vi "Initialise.vi"(8 "error in (no error)":errorcluster, 10 "Message in":refnum<class "InitialiseMessage.lvclass">, 11 "DAQCascade512 in":refnum<class "DAQCascade512.lvclass">) -> (0 "error out":errorcluster, 3 "DAQCascade512 out":refnum<class "DAQCascade512.lvclass">)   [LabVIEW 2012, in "DAQCascade512.lvclass"]
doc: "This method is called when an initialise message is received. It mainly initialises the RabbitMQ connectivity. \n\nOverride this method when your component needs special initialisation (e.g. of software or hardware resources). In that case, don't forget to call the parent for proper implementation. If your component owns subcomponents, they count as resources, so you have to initialise them by calling their own initialise functions"
uses:
  DAQCascade512.lvclass
  <vilib>/Distrio/Murmex/InitialiseMessage/InitialiseMessage.lvclass
  <vilib>/Distrio/Murmex/Murmex/Murmex.lvclass
  DAQCascade512.lvclass/DAQCascade512.ctl
panel:
  # "This method is called when the INTIALISE\ntrigger is sent. \n\nOverride this method when your component needs to\nrespond to this trigger. \n\nCall parent for proper implementation"
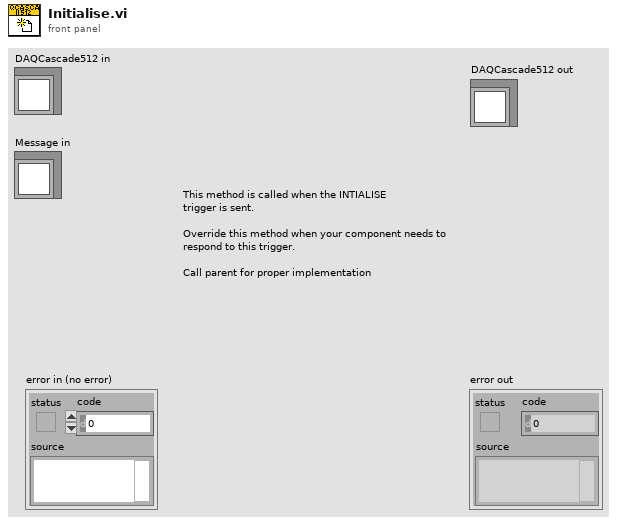
[diagram p1: front panel]
types:
  T1 = typedef "Image_type.ctl" = u32
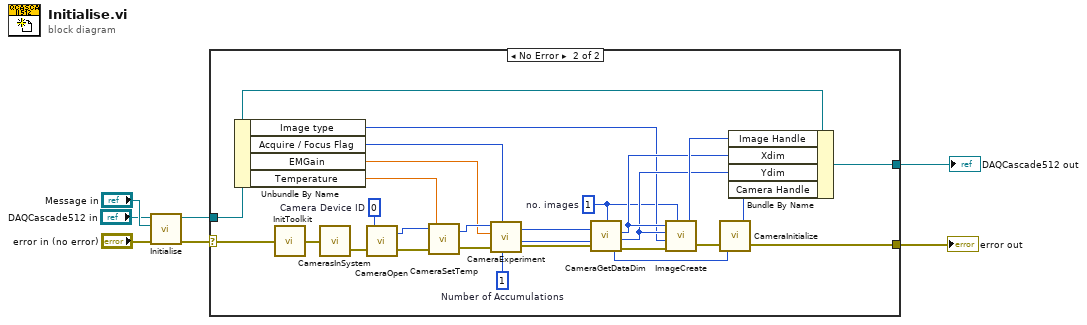
[diagram p0: block diagram]
diagram:
  n1 = call-parent "Initialise.vi"("error in (no error)"="error in (no error)", "Message in"="Message in", "Murmex in"="DAQCascade512 in") -> ("error out"=w4:errorcluster, "Murmex out"=w2:refnum<class "DAQCascade512.lvclass">)  [unwired: 7 in]
  n2 = case shown="No Error" w4 {
    selector: w4 -> [w9 w15]
    tunnel: [w9 w14] -> w3
    tunnel: w2 -> [w8 w13]
    tunnel: [w8 w11] -> w1
    frame Error {
    }
    frame No Error {
      w10 = 1  # no. images
      w29 = u32 1  # Number of Accumulations
      w35 = u32 0  # Camera Device ID
      n3 = Unbundle By Name(w13) -> ("Image type"=w16:T1, "Acquire / Focus Flag"=w17:u32, "EMGain"=w18:dbl, "Temperature"=w19:dbl)
      n4 = call <userlib>:"InitToolkit.vi"("error in"=w15) -> ("error out"=w25:errorcluster)
      n5 = call <userlib>:"CamerasInSystem.vi"("error in"=w25) -> ("error out"=w30:errorcluster)  [unwired: 1 out]
      n6 = call <userlib>:"CameraOpen.vi"("error in"=w30, "Camera Device ID"=w35) -> ("error out"=w33:errorcluster, "Camera Handle"=w34:u32)
      n7 = call <userlib>:"CameraSetTemp.vi"("error in (no error)"=w33, "Temperature"=w19, "Camera Handle"=w34) -> ("error out"=w24:errorcluster, "Camera Handle"=w23:u32)
      n8 = call <userlib>:"CameraExperiment.vi"("Number of Accumulations"=w29, "Acquire / Focus Flag"=w17, "error in"=w24, "Number of Images"=w10, "Exposure (sec)"=w18, "Camera Handle"=w23) -> ("error out"=w32:errorcluster, "Camera Handle"=w27:u32)
      n9 = call <userlib>:"CameraGetDataDim.vi"("Camera Handle"=w27, "error in"=w32) -> ("Camera Handle"=w26:u32, "Xdim"=w21:u32, "Ydim"=w20:u32, "error out"=w31:errorcluster)
      n10 = call <userlib>:"ImageCreate.vi"("X dimension"=w21, "Y dimension"=w20, "Data Type"=w16, "error in"=w31, "Number Of Frames"=w10) -> ("Image Handle"=w22:u32, "error out"=w28:errorcluster)
      n11 = call <userlib>:"CameraInitialize.vi"("error in"=w28, "Camera Handle"=w26) -> ("error out"=w14:errorcluster, "Camera Handle"=w12:u32)
      n12 = Bundle By Name(cluster=w13, "Image Handle"=w22, "Xdim"=w21, "Ydim"=w20, "Camera Handle"=w12) -> (w11:refnum<class "DAQCascade512.lvclass">)
    }
  }
  "error out" <- w3
  "DAQCascade512 out" <- w1
